vi "CRYAlign Ref Check.vi"(6 "Align Reference":cluster{dbl, dbl}={1250.0, 4.5} {"?" format="%.1f"}, 7 "Limits":u16(ring)=2 items=["Upper Only", "Lower Only", "Upper & Lower"], 8 "Data":cluster{"Hz":dbl, "dB":dbl}[](array[cluster])=[{"Hz"=200.0, "dB"=2.9}, {"Hz"=500.0, "dB"=3.5}, {"Hz"=1000.0, "dB"=5.0}, {"Hz"=2000.0, "dB"=6.0}, {"Hz"=4500.0, "dB"=4.0}] {"dB" format="%.1f"}, 9 "Lower Limit":cluster{"Hz":dbl, "y":dbl}[](array[cluster])=[{"Hz"=400.0, "y"=0.5}, {"Hz"=1000.0, "y"=3.5}, {"Hz"=3000.0, "y"=1.5}] {"y" format="%.1f"}, 11 "Upper Limit":cluster{"Hz":dbl, "y":dbl}[](array[cluster])=[{"Hz"=300.0, "y"=4.0}, {"Hz"=1000.0, "y"=6.5}, {"Hz"=4000.0, "y"=5.0}, {"Hz"=5000.0, "y"=4.2}] {"y" format="%.1f"}) -> (1 "Align Flag":bool)   [LabVIEW 2013]
uses:
  CRYLimit edit global.vi
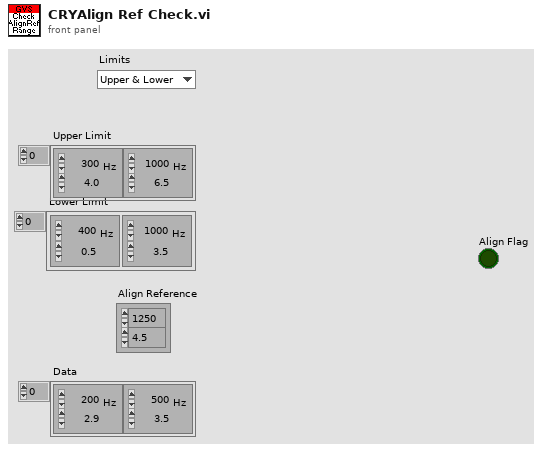
[diagram p1: front panel]
types:
  T1 = enum16{"OK", "Yes", "YesNo", "YesNoCancel", "ReplaceAppend"}
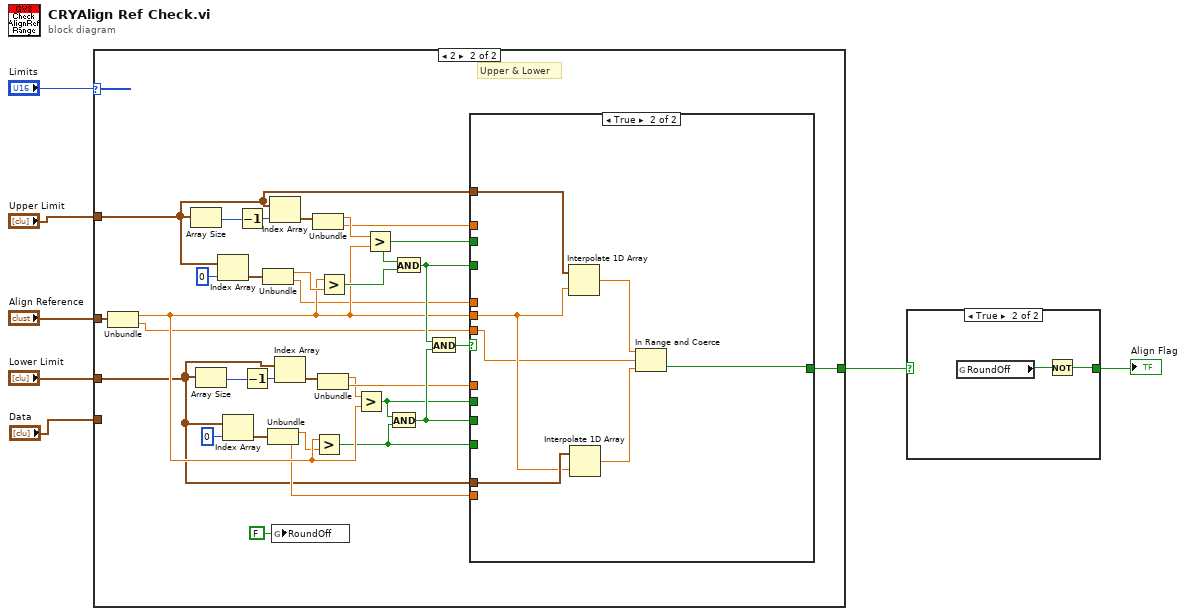
[diagram p0: block diagram]
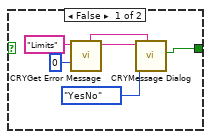
[diagram p2: hidden frame]
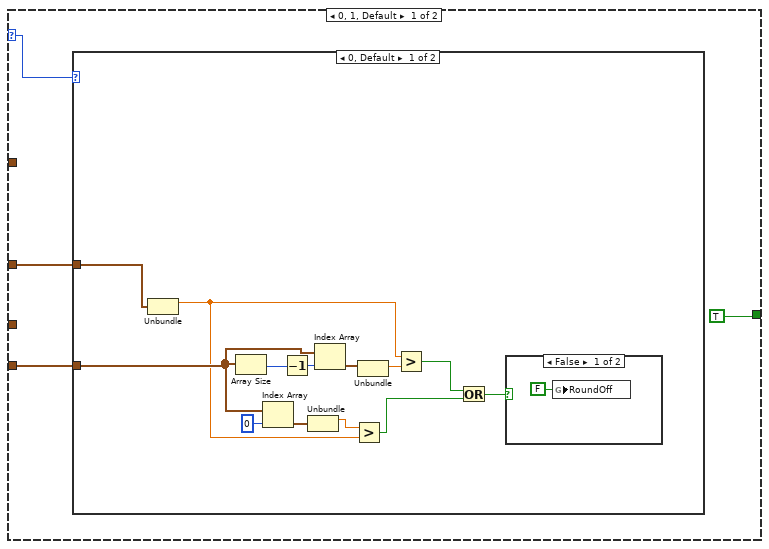
[diagram p3: hidden frame]
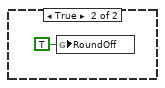
[diagram p4: hidden frame]
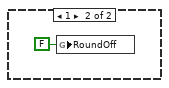
[diagram p5: hidden frame]
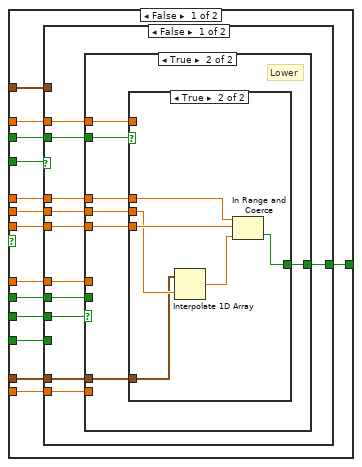
[diagram p6: hidden frame]
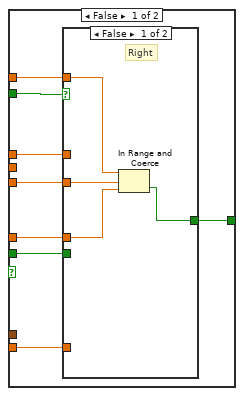
[diagram p7: hidden frame]
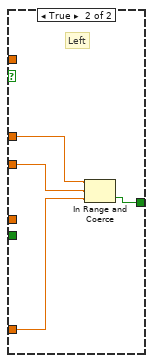
[diagram p8: hidden frame]
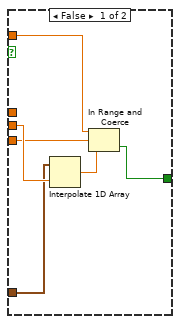
[diagram p9: hidden frame]
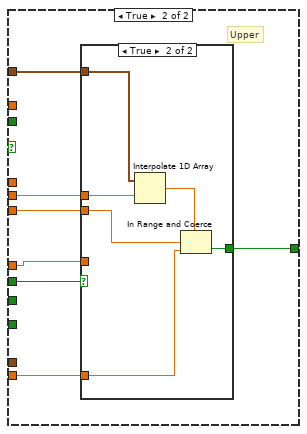
[diagram p10: hidden frame]
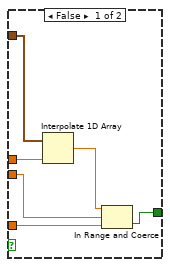
[diagram p11: hidden frame]
diagram:
  n1 = case shown="2" "Limits" {
    selector: "Limits" -> [w11 _]
    tunnel: "Upper Limit" -> [_ w34]
    tunnel: "Align Reference" -> [w10 w33]
    tunnel: "Lower Limit" -> [_ w32]
    tunnel: [TRUE w29] -> w2
    tunnel: "Data" -> [w9 _]
    frame 0, 1, Default {
      n2 = case shown="0, Default" w11 {
        tunnel: w10 -> [w19 _]
        tunnel: w9 -> [w18 _]
        frame 0, Default {
          n3 = Unbundle(w19) -> (w14:dbl)  [unwired: 1 out]
          n4 = Array Size(array=w18) -> (size(s)=w24:i32)
          n5 = Index Array(array=w18, index=0) -> (element=w20:cluster{"Hz":dbl, "dB":dbl})
          n6 = Decrement(x=w24) -> (x-1=w23:i32)
          n7 = Unbundle(w20) -> ("Hz"=w15:dbl)  [unwired: 1 out]
          n8 = Index Array(array=w18, index=w23) -> (element=w21:cluster{"Hz":dbl, "dB":dbl})
          n9 = Greater?(x=w15, y=w14) -> (0:w13:bool)
          n10 = Unbundle(w21) -> ("Hz"=w16:dbl)  [unwired: 1 out]
          n11 = Greater?(x=w14, y=w16) -> (0:w17:bool)
          n12 = Or(x=w17, y=w13) -> (x .or. y?=w12:bool)
          n13 = case shown="False" w12 {
            frame False {
              n14 = global write "CRYLimit edit global.vi" "RoundOff"(FALSE ("RoundOff")) -> ()
            }
            frame True {
              n15 = global write "CRYLimit edit global.vi" "RoundOff"(TRUE ("RoundOff")) -> ()
            }
          }
        }
        frame 1 {
          n16 = global write "CRYLimit edit global.vi" "RoundOff"(FALSE ("RoundOff")) -> ()
        }
      }
    }
    frame 2 {
      # "Upper & Lower"
      n17 = Unbundle(w33) -> (w43:dbl, w31:dbl)
      n18 = Array Size(array=w34) -> (size(s)=w59:i32)
      n19 = Array Size(array=w32) -> (size(s)=w51:i32)
      n20 = Index Array(array=w34, index=0) -> (element=w55:cluster{"Hz":dbl, "y":dbl})
      n21 = Index Array(array=w32, index=0) -> (element=w47:cluster{"Hz":dbl, "y":dbl})
      n22 = Decrement(x=w59) -> (x-1=w58:i32)
      n23 = Decrement(x=w51) -> (x-1=w50:i32)
      n24 = Unbundle(w55) -> ("Hz"=w53:dbl, "y"=w36:dbl)
      n25 = Unbundle(w47) -> ("Hz"=w40:dbl, "y"=w39:dbl)
      n26 = Index Array(array=w34, index=w58) -> (element=w56:cluster{"Hz":dbl, "y":dbl})
      n27 = global write "CRYLimit edit global.vi" "RoundOff"(FALSE ("RoundOff")) -> ()
      n28 = Index Array(array=w32, index=w50) -> (element=w48:cluster{"Hz":dbl, "y":dbl})
      n29 = Unbundle(w56) -> ("Hz"=w54:dbl, "y"=w35:dbl)
      n30 = Greater?(x=w43, y=w40) -> (0:w41:bool)
      n31 = Unbundle(w48) -> ("Hz"=w30:dbl, "y"=w38:dbl)
      n32 = Greater?(x=w43, y=w53) -> (0:w52:bool)
      n33 = Greater?(x=w30, y=w43) -> (0:w42:bool)
      n34 = Greater?(x=w54, y=w43) -> (0:w37:bool)
      n35 = And(x=w42, y=w41) -> (x .and. y?=w44:bool)
      n36 = And(x=w37, y=w52) -> (x .and. y?=w45:bool)
      n37 = And(x=w45, y=w44) -> (x .and. y?=w46:bool)
      n38 = case shown="True" w46 {
        tunnel: [w65 w139] -> w29
        tunnel: w45 -> [w73 _]
        tunnel: w44 -> [w72 _]
        tunnel: w43 -> [w67 w143]
        tunnel: w34 -> [w66 w145]
        tunnel: w32 -> [w61 w144]
        tunnel: w42 -> [w71 _]
        tunnel: w41 -> [w70 _]
        tunnel: w31 -> [w69 w142]
        tunnel: w39 -> [w68 _]
        tunnel: w38 -> [w64 _]
        tunnel: w37 -> [w63 _]
        tunnel: w36 -> [w62 _]
        tunnel: w35 -> [w60 _]
        frame False {
          n39 = case shown="False" w73 {
            tunnel: w72 -> [w84 _]
            tunnel: w71 -> [w76 w126]
            tunnel: w70 -> [_ _]
            tunnel: w69 -> [w80 w124]
            tunnel: w68 -> [w75 w121]
            tunnel: w67 -> [w81 w122]
            tunnel: w66 -> [_ w125]
            tunnel: [w78 w123] -> w65
            tunnel: w64 -> [w74 w120]
            tunnel: w63 -> [w83 _]
            tunnel: w62 -> [w82 _]
            tunnel: w61 -> [w79 _]
            tunnel: w60 -> [w77 _]
            frame False {
              n40 = case shown="True" w84 {
                tunnel: w83 -> [w92 w107]
                tunnel: w82 -> [w91 w106]
                tunnel: w81 -> [_ w105]
                tunnel: w80 -> [w88 w104]
                tunnel: w79 -> [_ w103]
                tunnel: [w87 w102] -> w78
                tunnel: w77 -> [w85 w101]
                tunnel: w76 -> [w90 _]
                tunnel: w75 -> [w89 _]
                tunnel: w74 -> [w86 _]
                frame False {
                  n41 = case shown="False" w92 {
                    tunnel: w91 -> [_ w100]
                    tunnel: w90 -> [_ _]
                    tunnel: w89 -> [_ w98]
                    tunnel: w88 -> [w94 w99]
                    tunnel: [w93 w97] -> w87
                    tunnel: w86 -> [w95 _]
                    tunnel: w85 -> [w96 _]
                    frame False {
                      # "Right"
                      n42 = In Range and Coerce(upper limit=w96, x=w94, lower limit=w95) -> (In Range?=w93:bool)  [unwired: 1 out]
                    }
                    frame True {
                      # "Left"
                      n43 = In Range and Coerce(upper limit=w100, x=w99, lower limit=w98) -> (In Range?=w97:bool)  [unwired: 1 out]
                    }
                  }
                }
                frame True {
                  # "Lower"
                  n44 = case shown="True" w107 {
                    tunnel: w106 -> [_ w119]
                    tunnel: w105 -> [w113 w116]
                    tunnel: w104 -> [w110 w118]
                    tunnel: w103 -> [w112 w115]
                    tunnel: [w108 w114] -> w102
                    tunnel: w101 -> [w109 _]
                    frame False {
                      n45 = Interpolate 1D Array(1:w113, 2:w112) -> (0:w111:dbl)
                      n46 = In Range and Coerce(upper limit=w109, x=w110, lower limit=w111) -> (In Range?=w108:bool)  [unwired: 1 out]
                    }
                    frame True {
                      n47 = Interpolate 1D Array(1:w116, 2:w115) -> (0:w117:dbl)
                      n48 = In Range and Coerce(upper limit=w119, x=w118, lower limit=w117) -> (In Range?=w114:bool)  [unwired: 1 out]
                    }
                  }
                }
              }
            }
            frame True {
              # "Upper"
              n49 = case shown="True" w126 {
                tunnel: w121 -> [_ w133]
                tunnel: w122 -> [w131 w138]
                tunnel: w125 -> [w130 w137]
                tunnel: w124 -> [w132 w135]
                tunnel: [w128 w134] -> w123
                tunnel: w120 -> [w127 _]
                frame False {
                  n50 = Interpolate 1D Array(1:w131, 2:w130) -> (0:w129:dbl)
                  n51 = In Range and Coerce(upper limit=w129, x=w132, lower limit=w127) -> (In Range?=w128:bool)  [unwired: 1 out]
                }
                frame True {
                  n52 = Interpolate 1D Array(1:w138, 2:w137) -> (0:w136:dbl)
                  n53 = In Range and Coerce(upper limit=w136, x=w135, lower limit=w133) -> (In Range?=w134:bool)  [unwired: 1 out]
                }
              }
            }
          }
        }
        frame True {
          n54 = Interpolate 1D Array(1:w143, 2:w145) -> (0:w141:dbl)
          n55 = Interpolate 1D Array(1:w143, 2:w144) -> (0:w140:dbl)
          n56 = In Range and Coerce(upper limit=w141, x=w142, lower limit=w140) -> (In Range?=w139:bool)  [unwired: 1 out]
        }
      }
    }
  }
  n57 = case shown="True" w2 {
    tunnel: [w146 w152] -> w3
    frame False {
      n58 = call "CRYGet Error Message.vi"("Error No"=0, "Kind"="Limits") -> ("Message"=w149:string, "Window Title"=w148:string)  [unwired: 4 in, 4 out]
      n59 = call "CRYMessage Dialog.vi"("Window Title"=w148, "YesNoCancel"=T1."YesNo", "Message Content"=w149) -> ("YesNo"=w146:bool)  [unwired: 7 in, 1 out]
    }
    frame True {
      n60 = global read "CRYLimit edit global.vi" "RoundOff"() -> (w153:bool)
      n61 = Not(x=w153) -> (.not. x?=w152:bool)
    }
  }
  "Align Flag" <- w3
